vi "Pressure Flow Analysis.vi"(7 "Error In":errorcluster, 9 "Current File Path IN":path, 10 "Signals":dynamicdata(graph)) -> (0 "Error Out":errorcluster, 2 "Current File Path":path, 3 "Data cluster":T1)   [LabVIEW 2019, in "MainVIs.lvlib"]
uses:
  MainVIs.lvlib
  Controls/Save Data Cluster.ctl
  <vilib>/Analysis/baseanly.llb/Mean (DBL).vi
  <vilib>/Waveform/WDTOps.llb/WDT Get Waveform Subset DBL.vi
  <vilib>/Analysis/NI_AALBase.lvlib
  SubVIs.lvlib
panel:
  out "Section CQ":dbl
  out "Mean CQ":dbl format="%#_5g"
  out "Section SupraGP":dbl format="%#.4g"
  out "Section F0 (EGG)":dbl format="%#.3g"
  out "Mean F0 (EGG)":dbl format="%#.3g"
  out "Mean SupraGP":dbl format="%#.4g"
  out "Mean VE":dbl format="%#.3g"
  out "Mean SPL":dbl format="%#.3g"
  out "Mean F0":dbl format="%#.3g"
  out "Section VE":dbl format="%#.3g"
  out "Section SPL":dbl format="%#.3g"
  out "Section F0":dbl format="%#.3g"
  out "Section Flow":dbl format="%#.4g"
  out "Section SubGP":dbl format="%#.4g"
  in  "Mark Section":bool
  out "Sections Marked":i32
  in  "OK Button":bool
  out "Mean Flow":dbl format="%#.4g"
  out "Mean SubGP":dbl format="%#.4g"
  out "Data Trace (Expanded)":dynamicdata(graph)
  out "Data Trace":dynamicdata(graph)
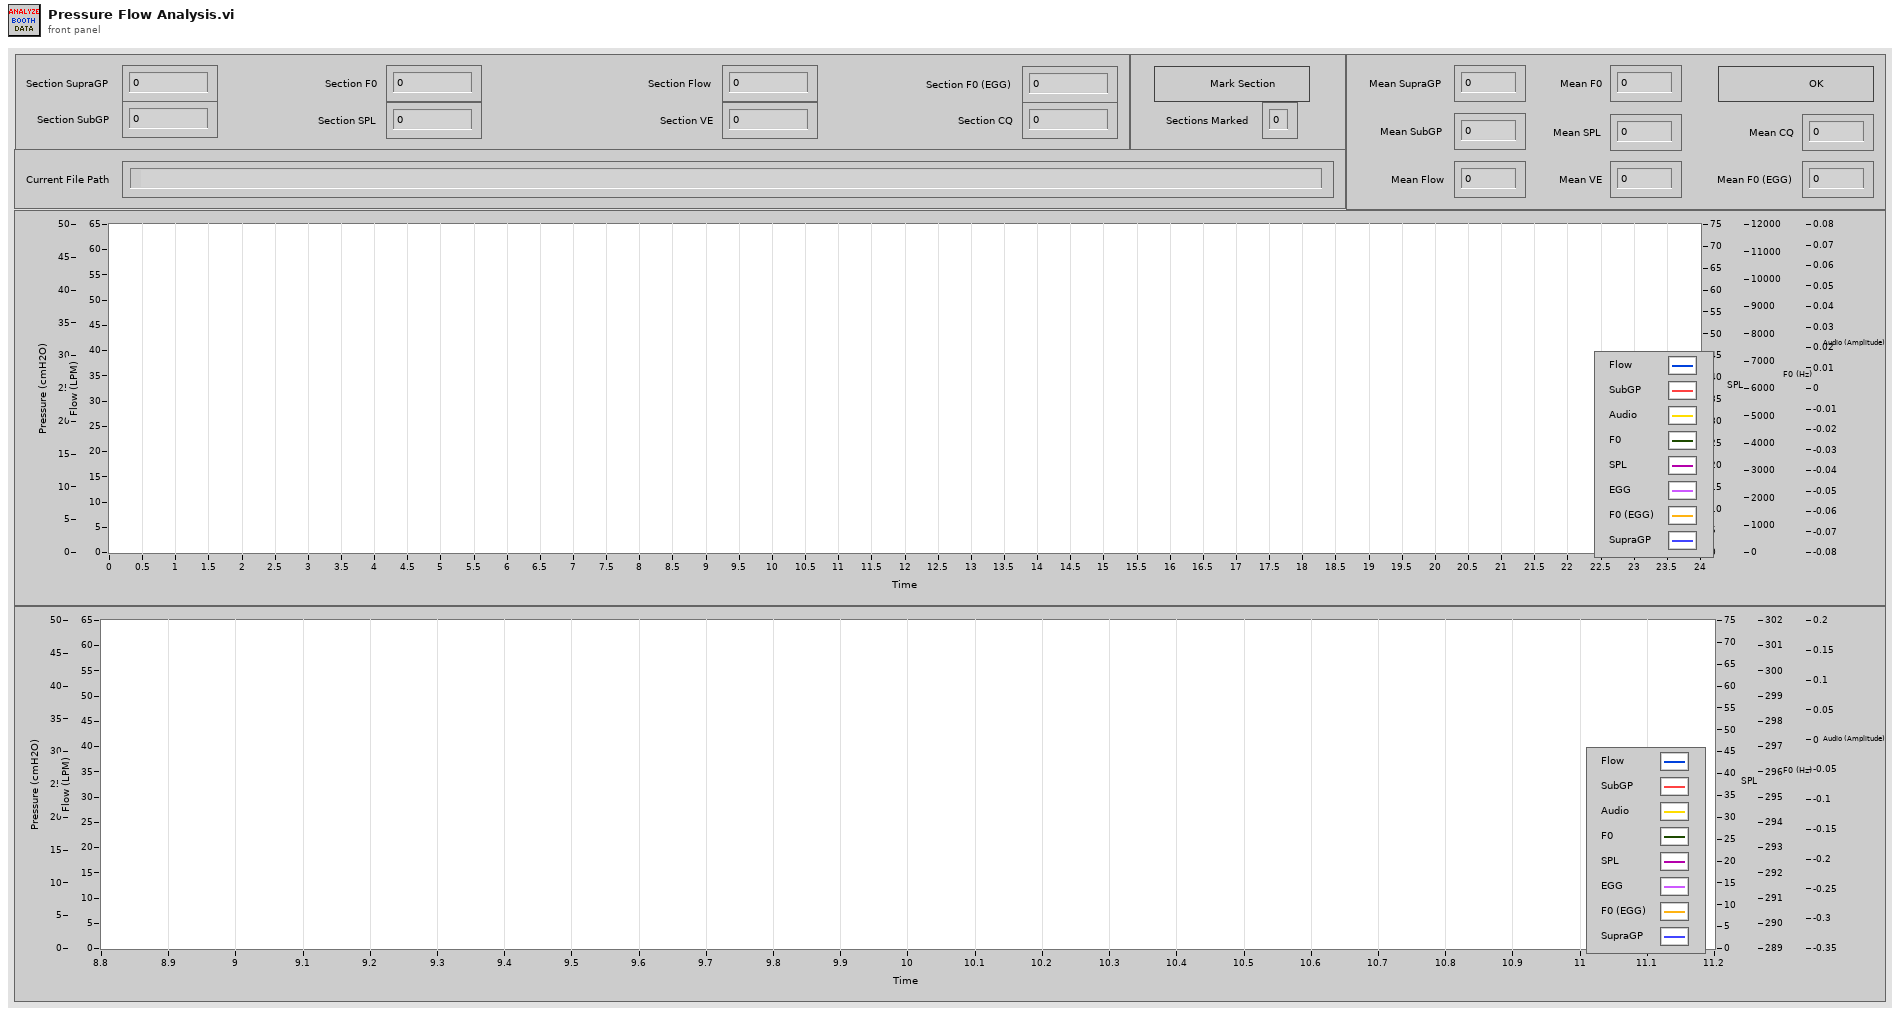
[diagram p1: front panel]
types:
  T1 = typedef "Save Data Cluster.ctl" = cluster{"Mean Flow":dbl, "Mean SubGP":dbl, "Mean SupraGP":dbl, "Mean F0":dbl, "Mean F0 (EGG)":dbl, "Mean VE":dbl, "Mean SPL":dbl, "Mean CQ":dbl, "Flow Array":dbl[], "SubGP Array":dbl[], "SupraGP Array":dbl[], "F0 Array":dbl[], "F0 (EGG) Array":dbl[], "VE Array":dbl[], "SPL Array":dbl[], "CQ Array":dbl[], "Times Array":dbl[][]}
  T2 = cluster{"Name":string, "Color":u32, "Style":u8, "Point Style":u8, "Name Visible":bool, "Allow Drag":bool, "Cursor Mode":u32, "Plot":i32, "Index":i32, "Position":cluster{"X":dbl, "Y":dbl}, "X Scale":u32, "Y Scale":u32, "Watch Plots":i32[], "Watch All Plots":bool, "Plot Area":i32, "Label Offset":cluster{"X":dbl, "Y":dbl}}[]
  T3 = cluster{"Updated List[0]":cluster{"Name":string, "Color":u32, "Style":u8, "Point Style":u8, "Name Visible":bool, "Allow Drag":bool, "Cursor Mode":u32, "Plot":i32, "Index":i32, "Position":cluster{"X":dbl, "Y":dbl}, "X Scale":u32, "Y Scale":u32, "Watch Plots":i32[], "Watch All Plots":bool, "Plot Area":i32, "Label Offset":cluster{"X":dbl, "Y":dbl}}, "Updated List[1]":cluster{"Name":string, "Color":u32, "Style":u8, "Point Style":u8, "Name Visible":bool, "Allow Drag":bool, "Cursor Mode":u32, "Plot":i32, "Index":i32, "Position":cluster{"X":dbl, "Y":dbl}, "X Scale":u32, "Y Scale":u32, "Watch Plots":i32[], "Watch All Plots":bool, "Plot Area":i32, "Label Offset":cluster{"X":dbl, "Y":dbl}}, "Updated List[2]":cluster{"Name":string, "Color":u32, "Style":u8, "Point Style":u8, "Name Visible":bool, "Allow Drag":bool, "Cursor Mode":u32, "Plot":i32, "Index":i32, "Position":cluster{"X":dbl, "Y":dbl}, "X Scale":u32, "Y Scale":u32, "Watch Plots":i32[], "Watch All Plots":bool, "Plot Area":i32, "Label Offset":cluster{"X":dbl, "Y":dbl}}, "Updated List[3]":cluster{"Name":string, "Color":u32, "Style":u8, "Point Style":u8, "Name Visible":bool, "Allow Drag":bool, "Cursor Mode":u32, "Plot":i32, "Index":i32, "Position":cluster{"X":dbl, "Y":dbl}, "X Scale":u32, "Y Scale":u32, "Watch Plots":i32[], "Watch All Plots":bool, "Plot Area":i32, "Label Offset":cluster{"X":dbl, "Y":dbl}}, "Updated List[4]":cluster{"Name":string, "Color":u32, "Style":u8, "Point Style":u8, "Name Visible":bool, "Allow Drag":bool, "Cursor Mode":u32, "Plot":i32, "Index":i32, "Position":cluster{"X":dbl, "Y":dbl}, "X Scale":u32, "Y Scale":u32, "Watch Plots":i32[], "Watch All Plots":bool, "Plot Area":i32, "Label Offset":cluster{"X":dbl, "Y":dbl}}, "Updated List[5]":cluster{"Name":string, "Color":u32, "Style":u8, "Point Style":u8, "Name Visible":bool, "Allow Drag":bool, "Cursor Mode":u32, "Plot":i32, "Index":i32, "Position":cluster{"X":dbl, "Y":dbl}, "X Scale":u32, "Y Scale":u32, "Watch Plots":i32[], "Watch All Plots":bool, "Plot Area":i32, "Label Offset":cluster{"X":dbl, "Y":dbl}}, "Updated List[6]":cluster{"Name":string, "Color":u32, "Style":u8, "Point Style":u8, "Name Visible":bool, "Allow Drag":bool, "Cursor Mode":u32, "Plot":i32, "Index":i32, "Position":cluster{"X":dbl, "Y":dbl}, "X Scale":u32, "Y Scale":u32, "Watch Plots":i32[], "Watch All Plots":bool, "Plot Area":i32, "Label Offset":cluster{"X":dbl, "Y":dbl}}, "Updated List[7]":cluster{"Name":string, "Color":u32, "Style":u8, "Point Style":u8, "Name Visible":bool, "Allow Drag":bool, "Cursor Mode":u32, "Plot":i32, "Index":i32, "Position":cluster{"X":dbl, "Y":dbl}, "X Scale":u32, "Y Scale":u32, "Watch Plots":i32[], "Watch All Plots":bool, "Plot Area":i32, "Label Offset":cluster{"X":dbl, "Y":dbl}}, "Updated List[8]":cluster{"Name":string, "Color":u32, "Style":u8, "Point Style":u8, "Name Visible":bool, "Allow Drag":bool, "Cursor Mode":u32, "Plot":i32, "Index":i32, "Position":cluster{"X":dbl, "Y":dbl}, "X Scale":u32, "Y Scale":u32, "Watch Plots":i32[], "Watch All Plots":bool, "Plot Area":i32, "Label Offset":cluster{"X":dbl, "Y":dbl}}}
  T4 = typedef "LVCursorListTypeDef.ctl" = cluster{"Name":string, "Color":u32, "Style":u8, "Point Style":u8, "Name Visible":bool, "Allow Drag":bool, "Cursor Mode":u32, "Plot":i32, "Index":i32, "Position":cluster{"X":dbl, "Y":dbl}, "X Scale":u32, "Y Scale":u32, "Watch Plots":i32[], "Watch All Plots":bool, "Plot Area":i32, "Label Offset":cluster{"X":dbl, "Y":dbl}}[]
  T5 = cluster{"CrsrList[0]":cluster{"Name":string, "Color":u32, "Style":u8, "Point Style":u8, "Name Visible":bool, "Allow Drag":bool, "Cursor Mode":u32, "Plot":i32, "Index":i32, "Position":cluster{"X":dbl, "Y":dbl}, "X Scale":u32, "Y Scale":u32, "Watch Plots":i32[], "Watch All Plots":bool, "Plot Area":i32, "Label Offset":cluster{"X":dbl, "Y":dbl}}, "CrsrList[1]":cluster{"Name":string, "Color":u32, "Style":u8, "Point Style":u8, "Name Visible":bool, "Allow Drag":bool, "Cursor Mode":u32, "Plot":i32, "Index":i32, "Position":cluster{"X":dbl, "Y":dbl}, "X Scale":u32, "Y Scale":u32, "Watch Plots":i32[], "Watch All Plots":bool, "Plot Area":i32, "Label Offset":cluster{"X":dbl, "Y":dbl}}, "CrsrList[2]":cluster{"Name":string, "Color":u32, "Style":u8, "Point Style":u8, "Name Visible":bool, "Allow Drag":bool, "Cursor Mode":u32, "Plot":i32, "Index":i32, "Position":cluster{"X":dbl, "Y":dbl}, "X Scale":u32, "Y Scale":u32, "Watch Plots":i32[], "Watch All Plots":bool, "Plot Area":i32, "Label Offset":cluster{"X":dbl, "Y":dbl}}, "CrsrList[3]":cluster{"Name":string, "Color":u32, "Style":u8, "Point Style":u8, "Name Visible":bool, "Allow Drag":bool, "Cursor Mode":u32, "Plot":i32, "Index":i32, "Position":cluster{"X":dbl, "Y":dbl}, "X Scale":u32, "Y Scale":u32, "Watch Plots":i32[], "Watch All Plots":bool, "Plot Area":i32, "Label Offset":cluster{"X":dbl, "Y":dbl}}, "CrsrList[4]":cluster{"Name":string, "Color":u32, "Style":u8, "Point Style":u8, "Name Visible":bool, "Allow Drag":bool, "Cursor Mode":u32, "Plot":i32, "Index":i32, "Position":cluster{"X":dbl, "Y":dbl}, "X Scale":u32, "Y Scale":u32, "Watch Plots":i32[], "Watch All Plots":bool, "Plot Area":i32, "Label Offset":cluster{"X":dbl, "Y":dbl}}, "CrsrList[5]":cluster{"Name":string, "Color":u32, "Style":u8, "Point Style":u8, "Name Visible":bool, "Allow Drag":bool, "Cursor Mode":u32, "Plot":i32, "Index":i32, "Position":cluster{"X":dbl, "Y":dbl}, "X Scale":u32, "Y Scale":u32, "Watch Plots":i32[], "Watch All Plots":bool, "Plot Area":i32, "Label Offset":cluster{"X":dbl, "Y":dbl}}, "CrsrList[6]":cluster{"Name":string, "Color":u32, "Style":u8, "Point Style":u8, "Name Visible":bool, "Allow Drag":bool, "Cursor Mode":u32, "Plot":i32, "Index":i32, "Position":cluster{"X":dbl, "Y":dbl}, "X Scale":u32, "Y Scale":u32, "Watch Plots":i32[], "Watch All Plots":bool, "Plot Area":i32, "Label Offset":cluster{"X":dbl, "Y":dbl}}, "CrsrList[7]":cluster{"Name":string, "Color":u32, "Style":u8, "Point Style":u8, "Name Visible":bool, "Allow Drag":bool, "Cursor Mode":u32, "Plot":i32, "Index":i32, "Position":cluster{"X":dbl, "Y":dbl}, "X Scale":u32, "Y Scale":u32, "Watch Plots":i32[], "Watch All Plots":bool, "Plot Area":i32, "Label Offset":cluster{"X":dbl, "Y":dbl}}, "CrsrList[8]":cluster{"Name":string, "Color":u32, "Style":u8, "Point Style":u8, "Name Visible":bool, "Allow Drag":bool, "Cursor Mode":u32, "Plot":i32, "Index":i32, "Position":cluster{"X":dbl, "Y":dbl}, "X Scale":u32, "Y Scale":u32, "Watch Plots":i32[], "Watch All Plots":bool, "Plot Area":i32, "Label Offset":cluster{"X":dbl, "Y":dbl}}}
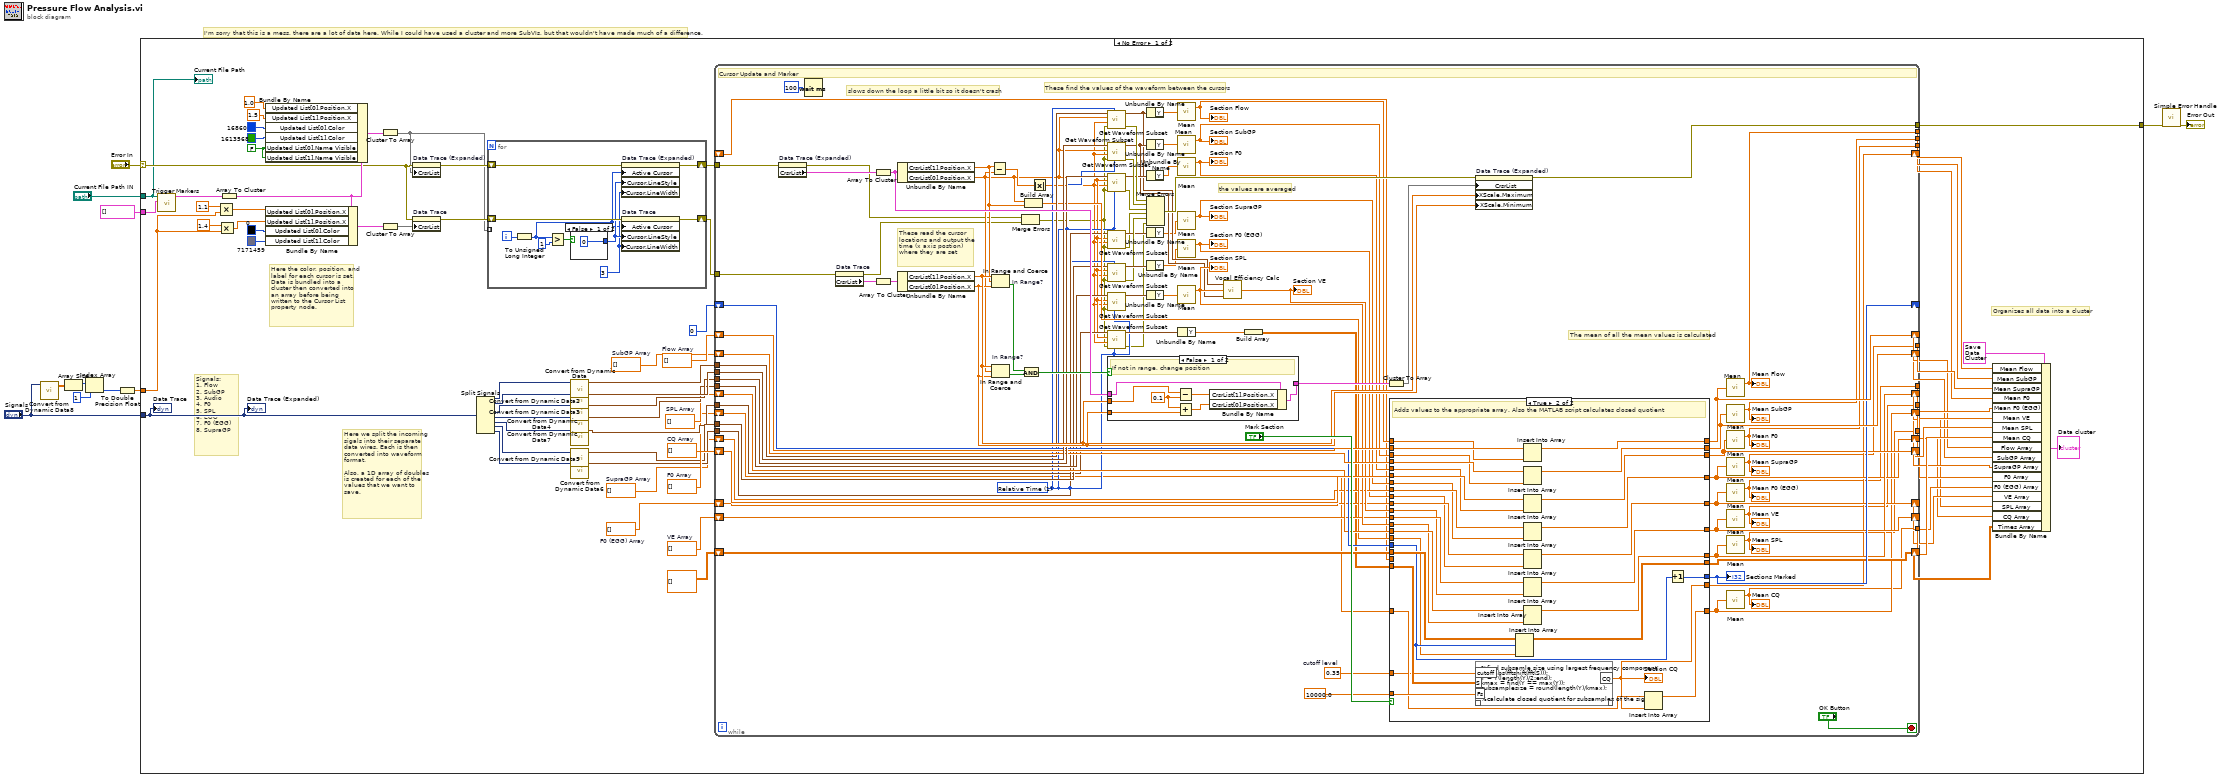
[diagram p0: block diagram]
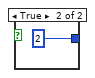
[diagram p2: hidden frame]
diagram:
  # "I'm sorry that this is a mess, there are a lot of data here. While I could have used a cluster and more SubVIs, but that wouldn't have made much of a difference."
  n1 = call "Convert from Dynamic Data8"("Dynamic Data Type"="Signals") -> ("Array"=w5:dbl[][])  [unwired: 3 in]
  n2 = Array Size(array=w5) -> (size(s)=w4:i32[])
  n3 = Index Array(array=w4, index=1) -> (element=w2:i32)
  n4 = To Double Precision Float(number=w2) -> (double precision float=w1:dbl)
  n5 = case shown="No Error" "Error In" {
    selector: "Error In" -> [w61 w239]
    tunnel: [w60 w239] -> w10
    tunnel: "Signals" -> [w81 _]
    tunnel: T2 [] ("Cursor List") -> [w24 _]
    tunnel: "Current File Path IN" -> [w25 _]
    tunnel: w1 -> [w12 _]
    frame No Error {
      w45 = dbl[] []  # CQ Array
      w49 = dbl[] []  # F0 (EGG) Array
      w48 = dbl[] []  # SupraGP Array
      w55 = FALSE ("Cursor List[1].Name Visible")
      w57 = dbl[] []  # VE Array
      w56 = dbl[] []  # SPL Array
      w64 = dbl[] []  # Flow Array
      w62 = dbl[] []  # F0 Array
      w63 = dbl[] []  # SubGP Array
      # "Here we split the incoming sigals into their separate data wires. Each is then converted into waveform format.\n\nAlso, a 1D array of doubles is created for each of the values that we want to save."
      # "Here the color, position, and label for each cursor is set. Data is bundled into a cluster then converted into an array before being written to the Cursor List property node."
      # "Organizes all data into a cluster"
      # "Signals:\n1. Flow\n2. SubGP\n3. Audio\n4. F0\n5. SPL \n6. EGG\n7. F0 (EGG)\n8. SupraGP"
      n6 = call "Trigger Markers.vi"("Cluster In"=w24, "Current File Path IN"=w25) -> ("Updated List"=w23:T2)  [unwired: 9 in]
      n7 = Multiply(x=1.1 ("Cursor List[0].Position.X"), y=w12) -> (x*y=w15:dbl)
      n8 = Multiply(x=1.4 ("Cursor List[1].Position.X"), y=w12) -> (x*y=w13:dbl)
      n9 = Array To Cluster(array=w23) -> (cluster=w69:T3)
      n10 = Bundle By Name(cluster=w69, "Updated List[0].Position.X"=1.0 ("Cursor List[0].Position.X"), "Updated List[1].Position.X"=1.5 ("Cursor List[0].Position.Y"), "Updated List[0].Color"=u32 16860, "Updated List[1].Color"=u32 1613568, "Updated List[0].Name Visible"=w55, "Updated List[1].Name Visible"=w55) -> (w76:T3)
      n11 = Bundle By Name(cluster=w69, "Updated List[0].Position.X"=w15, "Updated List[1].Position.X"=w13, "Updated List[0].Color"=u32 0, "Updated List[1].Color"=u32 7171459) -> (w77:T3)
      n12 = Cluster To Array(cluster=w76) -> (array=w17:T2)
      n13 = Cluster To Array(cluster=w77) -> (array=w18:T2)
      n14 = property on="Data Trace (Expanded)" class="WFGraph (strict)"(error in=w61, "CrsrList"=w17) -> (error out=w21:errorcluster)  [unwired: 1 in, 1 out]
      n15 = property on="Data Trace" class="WFGraph (strict)"(error in=w61, "CrsrList"=w18) -> (error out=w19:errorcluster)  [unwired: 1 in, 1 out]
      n16 = Split Signals(w81) -> (w80:dynamicdata, w79:dynamicdata, w78:dynamicdata, w59:dynamicdata, w47:dynamicdata, w53:dynamicdata, w52:dynamicdata)  [unwired: 8 in, 1 out]
      n17 = for {
        shift-right: [w91] -> w22
        shift-left: w21 -> [w90]
        shift-right: [w89] -> w20
        shift-left: w19 -> [w88]
        tunnel: w17 -> [_] mode=indexing
        i -> [w86]
        w83 = u8 3 ("Cursor.Line Width")
        n18 = To Unsigned Long Integer(number=w86) -> (unsigned 32bit integer=w82:u32)
        n19 = Greater?(x=w82, y=u32 1) -> (0:w84:bool)
        n20 = case shown="False" w84 {
          tunnel: [u8 0 ("Cursor.Line Style") u8 2 ("Cursor.Line Style")] -> w87
          frame False {
          }
          frame True {
          }
        }
        n21 = property on="Data Trace (Expanded)" class="WFGraph (strict)"(error in=w90, "Active Cursor"=w82, "Cursor.LineStyle"=w87, "Cursor.LineWidth"=w83) -> (error out=w91:errorcluster)  [unwired: 1 in, 1 out]
        n22 = property on="Data Trace" class="WFGraph (strict)"(error in=w88, "Active Cursor"=w82, "Cursor.LineStyle"=w87, "Cursor.LineWidth"=w83) -> (error out=w89:errorcluster)  [unwired: 1 in, 1 out]
      }
      n23 = call "Convert from Dynamic Data"("Dynamic Data Type"=w80) -> ("Waveform"=w68:waveform(dbl))  [unwired: 3 in]
      n24 = call "Convert from Dynamic Data2"("Dynamic Data Type"=w79) -> ("Waveform"=w67:waveform(dbl))  [unwired: 3 in]
      n25 = call "Convert from Dynamic Data3"("Dynamic Data Type"=w78) -> ("Waveform"=w66:waveform(dbl))  [unwired: 3 in]
      n26 = call "Convert from Dynamic Data4"("Dynamic Data Type"=w59) -> ("Waveform"=w58:waveform(dbl))  [unwired: 3 in]
      n27 = call "Convert from Dynamic Data7"("Dynamic Data Type"=w47) -> ("Waveform"=w46:waveform(dbl))  [unwired: 3 in]
      n28 = call "Convert from Dynamic Data5"("Dynamic Data Type"=w53) -> ("Waveform"=w51:waveform(dbl))  [unwired: 3 in]
      n29 = call "Convert from Dynamic Data6"("Dynamic Data Type"=w52) -> ("Waveform"=w50:waveform(dbl))  [unwired: 3 in]
      n30 = while {
        tunnel: w68 -> [w141]
        tunnel: w67 -> [w170]
        tunnel: w66 -> [w171]
        shift-right: [w154] -> _
        shift-left: 0 -> [w155]
        shift-right: [w153] -> w32
        shift-left: w62 -> [w160]
        shift-right: [w158] -> w34
        shift-left: w63 -> [w161]
        shift-right: [w157] -> w35
        shift-left: w64 -> [w159]
        tunnel: w20 -> [w183]
        tunnel: w22 -> [w182]
        tunnel: [w99] -> w60
        tunnel: w58 -> [w152]
        shift-right: [w145] -> w30
        shift-left: w57 -> [w147]
        shift-right: [w144] -> w29
        shift-left: w56 -> [w149]
        shift-right: [w136] -> w27
        shift-left: dbl[][] [] -> [w137]
        tunnel: w51 -> [w127]
        tunnel: w50 -> [w122]
        shift-right: [w131] -> w33
        shift-left: w48 -> [w133]
        shift-right: [w130] -> w31
        shift-left: w49 -> [w132]
        tunnel: w46 -> [w118]
        shift-right: [w111] -> _
        shift-left: _ -> [w94]
        shift-right: [w109] -> w28
        shift-left: w45 -> [w110]
        tunnel: [w108] -> w43
        tunnel: [w107] -> w42
        tunnel: [w106] -> w41
        tunnel: [w105] -> w40
        tunnel: [w104] -> w39
        tunnel: [w103] -> w38
        tunnel: [w102] -> w37
        tunnel: [w101] -> w36
        stop <- "OK Button" stop-if-true
        w100 = 0.35  # cutoff level
        w117 = u16 1 items=["Samples", "Relative Time"] ("start/duration format")
        # "The mean of all the mean values is calculated"
        # "the values are averaged"
        # "These find the values of the waveform between the cursors"
        # "These read the cursor locations and output the time (x axis postion) where they are set"
        # "slows down the loop a little bit so it doesn't crash"
        # "Cursor Update and Marker"
        n31 = property on="Data Trace (Expanded)" class="WFGraph (strict)"(error in=w182) -> (error out=w98:errorcluster, "CrsrList"=w185:T4)  [unwired: 1 in, 1 out]
        n32 = Wait (ms)(milliseconds to wait=u32 100) -> ()  [unwired: 1 out]
        n33 = property on="Data Trace" class="WFGraph (strict)"(error in=w183) -> (error out=w97:errorcluster, "CrsrList"=w184:T4)  [unwired: 1 in, 1 out]
        n34 = Array To Cluster(array=w185) -> (cluster=w178:T5)
        n35 = Array To Cluster(array=w184) -> (cluster=w181:T5)
        n36 = Unbundle By Name(w178) -> ("CrsrList[1].Position.X"=w134:dbl, "CrsrList[0].Position.X"=w116:dbl)
        n37 = Unbundle By Name(w181) -> ("CrsrList[1].Position.X"=w174:dbl, "CrsrList[0].Position.X"=w173:dbl)
        n38 = Subtract(x=w134, y=w116) -> (x-y=w172:dbl)
        n39 = In Range and Coerce "In Range?"(upper limit=w174, x=w134, lower limit=w173) -> (In Range?=w177:bool)  [unwired: 1 out]
        n40 = In Range and Coerce "In Range?"(upper limit=w174, x=w116, lower limit=w173) -> (In Range?=w176:bool)  [unwired: 1 out]
        n41 = Merge Errors(w98, w97) -> (w96:errorcluster)
        n42 = And(x=w177, y=w176) -> (x .and. y?=w175:bool)
        n43 = Build Array(w116, w134) -> (w135:dbl[])
        n44 = Absolute Value(x=w172) -> (abs(x)=w115:dbl)
        n45 = call-poly <vilib>:"Get Waveform Subset.vi"("start/duration format"=w117, "error in (no error)"=w96, "duration"=w115, "start samples/time"=w116, "waveform in"=w141) -> ("error out"=w169:errorcluster, "waveform out"=w139:waveform(dbl))  [unwired: 1 in, 2 out]
        n46 = call-poly <vilib>:"Get Waveform Subset.vi"("start/duration format"=w117, "error in (no error)"=w96, "duration"=w115, "start samples/time"=w116, "waveform in"=w170) -> ("error out"=w168:errorcluster, "waveform out"=w140:waveform(dbl))  [unwired: 1 in, 2 out]
        n47 = call-poly <vilib>:"Get Waveform Subset.vi"("start/duration format"=w117, "error in (no error)"=w96, "duration"=w115, "start samples/time"=w116, "waveform in"=w171) -> ("error out"=w167:errorcluster, "waveform out"=w163:waveform(dbl))  [unwired: 1 in, 2 out]
        n48 = call-poly <vilib>:"Get Waveform Subset.vi"("start/duration format"=w117, "error in (no error)"=w96, "duration"=w115, "start samples/time"=w116, "waveform in"=w122) -> ("error out"=w120:errorcluster, "waveform out"=w123:waveform(dbl))  [unwired: 1 in, 2 out]
        n49 = call-poly <vilib>:"Get Waveform Subset.vi"("start/duration format"=w117, "error in (no error)"=w96, "duration"=w115, "start samples/time"=w116, "waveform in"=w127) -> ("error out"=w126:errorcluster, "waveform out"=w128:waveform(dbl))  [unwired: 1 in, 2 out]
        n50 = call-poly <vilib>:"Get Waveform Subset.vi"("start/duration format"=w117, "error in (no error)"=w96, "duration"=w115, "start samples/time"=w116, "waveform in"=w152) -> ("waveform out"=w151:waveform(dbl))  [unwired: 1 in, 3 out]
        n51 = call-poly <vilib>:"Get Waveform Subset.vi"("start/duration format"=w117, "error in (no error)"=w96, "duration"=w115, "start samples/time"=w116, "waveform in"=w118) -> ("error out"=w95:errorcluster, "waveform out"=w119:waveform(dbl))  [unwired: 1 in, 2 out]
        n52 = case shown="False" w175 {
          tunnel: [w194 w195] -> w179
          tunnel: w178 -> [w193 w195]
          tunnel: w173 -> [w191 _]
          tunnel: w174 -> [w190 _]
          frame False {
            w192 = 0.1
            # "If not in range, change position"
            n53 = Subtract(x=w190, y=w192) -> (x-y=w189:dbl)
            n54 = Add(x=w192, y=w191) -> (x+y=w188:dbl)
            n55 = Bundle By Name(cluster=w193, "CrsrList[1].Position.X"=w189, "CrsrList[0].Position.X"=w188) -> (w194:T5)
          }
          frame True {
            # "Cursors are within bounds"
          }
        }
        n56 = Unbundle By Name(w139) -> ("Y"=w166:dbl[])
        n57 = Unbundle By Name(w140) -> ("Y"=w165:dbl[])
        n58 = Unbundle By Name(w163) -> ("Y"=w164:dbl[])
        n59 = Merge Errors(w169, w168, w167, w120, w126, w95) -> (w162:errorcluster)
        n60 = Unbundle By Name(w123) -> ("Y"=w124:dbl[])
        n61 = Unbundle By Name(w128) -> ("Y"=w129:dbl[])
        n62 = Unbundle By Name(w151) -> ("Y"=w150:dbl[])
        n63 = call-poly <vilib>:"Mean.vi"("X"=w166) -> ("mean"=w143:dbl)  [unwired: 1 out]
        "Section Flow" <- w143
        n64 = call-poly <vilib>:"Mean.vi"("X"=w165) -> ("mean"=w142:dbl)  [unwired: 1 out]
        "Section SubGP" <- w142
        n65 = call-poly <vilib>:"Mean.vi"("X"=w164) -> ("mean"=w156:dbl)  [unwired: 1 out]
        "Section F0" <- w156
        n66 = call-poly <vilib>:"Mean.vi"("X"=w124) -> ("mean"=w121:dbl)  [unwired: 1 out]
        "Section SupraGP" <- w121
        n67 = call-poly <vilib>:"Mean.vi"("X"=w129) -> ("mean"=w125:dbl)  [unwired: 1 out]
        "Section F0 (EGG)" <- w125
        n68 = call-poly <vilib>:"Mean.vi"("X"=w150) -> ("mean"=w148:dbl)  [unwired: 1 out]
        "Section SPL" <- w148
        n69 = Unbundle By Name(w119) -> ("Y"=w114:dbl[])
        n70 = call "Vocal Efficiency Calc.vi"("Pressure"=w140, "SPL"=w148, "Flow"=w139) -> ("Vocal Efficiency"=w146:dbl)  [unwired: 2 in]
        "Section VE" <- w146
        n71 = Build Array(w114) -> (w113:dbl[][])
        n72 = Cluster To Array(cluster=w179) -> (array=w180:T2)
        n73 = case shown="True" "Mark Section" {
          tunnel: w161 -> [w206 w238]
          tunnel: w160 -> [w205 w237]
          tunnel: w159 -> [w204 w236]
          tunnel: [w206 w235] -> w158
          tunnel: [w205 w234] -> w153
          tunnel: [w204 w233] -> w157
          tunnel: w143 -> [_ w232]
          tunnel: w142 -> [_ w231]
          tunnel: w156 -> [_ w230]
          tunnel: w155 -> [w203 w221]
          tunnel: [w203 w229] -> w154
          tunnel: w149 -> [w202 w228]
          tunnel: w148 -> [_ w227]
          tunnel: w147 -> [w201 w226]
          tunnel: [w202 w225] -> w144
          tunnel: [w201 w224] -> w145
          tunnel: w146 -> [_ w223]
          tunnel: w137 -> [w200 w222]
          tunnel: [w200 w220] -> w136
          tunnel: w135 -> [_ w219]
          tunnel: w133 -> [w199 w218]
          tunnel: w132 -> [w198 w217]
          tunnel: [w198 w216] -> w130
          tunnel: [w199 w215] -> w131
          tunnel: w125 -> [_ w214]
          tunnel: w121 -> [_ w213]
          tunnel: w113 -> [_ w212]
          tunnel: 10000.0 ("Real") -> [_ w211]
          tunnel: [w197 w208] -> w111
          tunnel: w94 -> [w197 _]
          tunnel: w110 -> [w196 w210]
          tunnel: [w196 w209] -> w109
          tunnel: w100 -> [_ w207]
          frame False {
            # "Waiting for \"Mark Section\" to be clicked"
          }
          frame True {
            # "Adds values to the appropriate array. Also the MATLAB script calculates closed quotient"
            n74 = script code="%find subsamle size using largest frequency component\nY = abs(fftshift(fft(S)));\nY = Y(length(Y)/2:end);\nkmax = find(Y == max(Y));\nsubsamplesize = round(length(Y)/kmax);\n\n%calculate closed quotient for subsamples of the signal, \n%then find the average for the whole signal\nsubsamples = ceil(length(S)/subsamplesize);\ncq = 0; %running total of closed quotient for each subsample\nfor i = 1:subsamples\n    starti = ((i-1)*subsamplesize)+1;\n    endi = i*subsamplesize;\n    if(endi <= length(S))\n        s = S(starti:endi);\n    else\n        s = S(starti:end);\n    end\n    minval = min(s);\n    s = s - minval;\n    maxval = max(s);\n    closed = length(find(s < (maxval*cutoff)));\n    cq = cq + (closed/length(s));\nend\n\n%calculate average closed quotient for whole signal\nCQ = cq/subsamples;\n\nfprintf(num2str(CQ));\nreturn;"("S"=w212, "Fs"=w211, "cutoff"=w207) -> ("CQ"=w208:dbl)  [unwired: 1 in, 1 out]
            "Section CQ" <- w208
            n75 = Insert Into Array(array=w222, index (row)=w221, new element=w219) -> (w220:dbl[][])  [unwired: 1 in]
            n76 = Insert Into Array(array=w236, new element=w232) -> (w233:dbl[])  [unwired: 1 in]
            n77 = Insert Into Array(array=w238, new element=w231) -> (w235:dbl[])  [unwired: 1 in]
            n78 = Insert Into Array(array=w237, new element=w230) -> (w234:dbl[])  [unwired: 1 in]
            n79 = Insert Into Array(array=w218, new element=w213) -> (w215:dbl[])  [unwired: 1 in]
            n80 = Insert Into Array(array=w217, new element=w214) -> (w216:dbl[])  [unwired: 1 in]
            n81 = Insert Into Array(array=w226, new element=w223) -> (w224:dbl[])  [unwired: 1 in]
            n82 = Insert Into Array(array=w228, new element=w227) -> (w225:dbl[])  [unwired: 1 in]
            n83 = Insert Into Array(array=w210, new element=w208) -> (w209:dbl[])  [unwired: 1 in]
            n84 = Increment(x=w221) -> (x+1=w229:i32)
          }
        }
        "Sections Marked" <- w154
        n85 = property on="Data Trace (Expanded)" class="WFGraph (strict)"(error in=w162, "CrsrList"=w180, "XScale.Maximum"=w174, "XScale.Minimum"=w173) -> (error out=w99:errorcluster)  [unwired: 1 in, 1 out]
        n86 = call-poly <vilib>:"Mean.vi"("X"=w157) -> ("mean"=w108:dbl)  [unwired: 1 out]
        "Mean Flow" <- w108
        n87 = call-poly <vilib>:"Mean.vi"("X"=w158) -> ("mean"=w107:dbl)  [unwired: 1 out]
        "Mean SubGP" <- w107
        n88 = call-poly <vilib>:"Mean.vi"("X"=w153) -> ("mean"=w105:dbl)  [unwired: 1 out]
        "Mean F0" <- w105
        n89 = call-poly <vilib>:"Mean.vi"("X"=w131) -> ("mean"=w106:dbl)  [unwired: 1 out]
        "Mean SupraGP" <- w106
        n90 = call-poly <vilib>:"Mean.vi"("X"=w130) -> ("mean"=w104:dbl)  [unwired: 1 out]
        "Mean F0 (EGG)" <- w104
        n91 = call-poly <vilib>:"Mean.vi"("X"=w145) -> ("mean"=w103:dbl)  [unwired: 1 out]
        "Mean VE" <- w103
        n92 = call-poly <vilib>:"Mean.vi"("X"=w144) -> ("mean"=w102:dbl)  [unwired: 1 out]
        "Mean SPL" <- w102
        n93 = call-poly <vilib>:"Mean.vi"("X"=w109) -> ("mean"=w101:dbl)  [unwired: 1 out]
        "Mean CQ" <- w101
      }
      n94 = Bundle By Name(cluster=T1 {"Mean Flow"=0.0, "Mean SubGP"=0.0, "Mean SupraGP"=0.0, "Mean F0"=0.0, "Mean F0 (EGG)"=0.0, "Mean VE"=0.0, "Mean SPL"=0.0, "Mean CQ"=0.0, "Flow Array"=[], "SubGP Array"=[], "SupraGP Array"=[], "F0 Array"=[], "F0 (EGG) Array"=[], "VE Array"=[], "SPL Array"=[], "CQ Array"=[], "Times Array"=[]} ("input cluster"), "Mean Flow"=w43, "Mean SubGP"=w42, "Mean SupraGP"=w41, "Mean F0"=w40, "Mean F0 (EGG)"=w39, "Mean VE"=w38, "Mean SPL"=w37, "Mean CQ"=w36, "Flow Array"=w35, "SubGP Array"=w34, "SupraGP Array"=w33, "F0 Array"=w32, "F0 (EGG) Array"=w31, "VE Array"=w30, "SPL Array"=w29, "CQ Array"=w28, "Times Array"=w27) -> (→"Data cluster":T1)
      "Data Trace" <- w81
      "Data Trace (Expanded)" <- w81
      "Current File Path" <- w25
    }
    frame Error {
    }
  }
  n95 = call <vilib>:"Simple Error Handler.vi"("error in (no error)"=w10) -> ("error out"=→"Error Out":errorcluster)  [unwired: 4 in, 4 out]
